vi "Confirm Assembly.vi"(8 "error in (no error)":errorcluster, 11 "Database Assembly in":refnum<class "Database Assembly.lvclass">) -> (0 "error out":errorcluster, 3 "Database Assembly out":refnum<class "Database Assembly.lvclass">)   [LabVIEW 2020, in "Database Assembly.lvclass"]
uses:
  Database Assembly.lvclass
  Module/Module.lvclass
  Database Assembly.lvclass/Database Assembly.ctl
panel:
  out "Array":refnum<class "Module.lvclass">[](array[class])
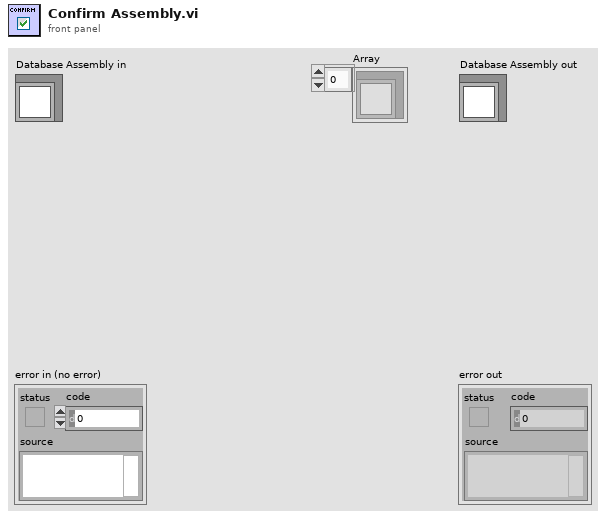
[diagram p1: front panel]
types:
  T1 = typedef "File Paths.ctl" = cluster{"Glue Pattern Folder":path, "Carrier Tray Folder":path, "Pick Up Tool Fixture Folder":path, "Components Folder":path, "Bellows Tool Offset.txt":path, "Pick Up Tool Offset.txt":path, "Dispense Tip Offset.txt":path, "Log Files":path, "Gantry Assembly Map.txt":path, "Syringe and offset map.txt":path}
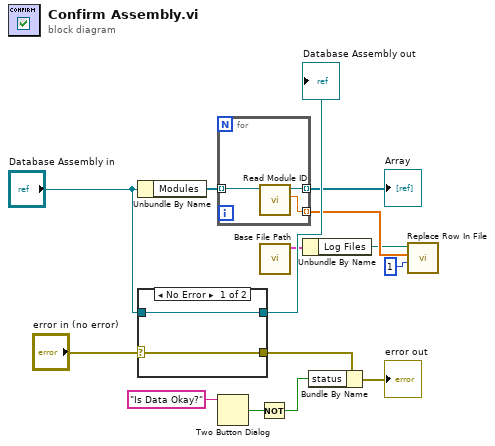
[diagram p0: block diagram]
diagram:
  n1 = Unbundle By Name("Database Assembly in") -> ("Modules"=w6:refnum<class "Module.lvclass">[])
  n2 = case shown="No Error" "error in (no error)" {
    selector: "error in (no error)" -> [w16 w18]
    tunnel: [w16 w18] -> w11
    tunnel: [w15 w17] -> w13
    tunnel: "Database Assembly in" -> [w15 w17]
    frame No Error {
    }
    frame Error {
    }
  }
  "Database Assembly out" <- w13
  n3 = for {
    tunnel: w6 -> [w21] mode=indexing
    tunnel: [w20] -> w4 mode=indexing
    tunnel: [w19] -> w5 mode=indexing
    n4 = call-dynamic "Read Module ID.vi"("Module in"=w21) -> ("Module ID"=w20:dbl, "Module out"=w19:refnum<class "Module.lvclass">)  [unwired: 8 in, 1 out]
  }
  "Array" <- w5
  n5 = Two Button Dialog(message="Is Data Okay?") -> (T button?=w10:bool)  [unwired: 2 in]
  n6 = Not(x=w10) -> (.not. x?=w9:bool)
  n7 = call "Base File Path.vi"() -> ("Paths Out"=w2:T1)  [unwired: 11 in]
  n8 = Unbundle By Name(w2) -> ("Log Files"=w1:path)
  n9 = Bundle By Name(cluster=w11, "status"=w9) -> (→"error out":errorcluster)
  n10 = call "Replace Row In File.vi"("Index"=1, "Insert Array"=w4, "Path"=w1) -> ()  [unwired: 8 in, 1 out]
